vi "Continued Fraction Complex.vi"(1 "b":cdb[](array[numeric]) format="%0.2f", 2 "a":cdb[](array[numeric]) format="%0.2f") -> (0 "result":cdb format="%0.2f")   [LabVIEW 2018, in "NI_Gmath.lvlib"]
uses:
  NI_Gmath.lvlib
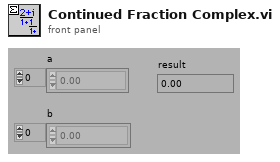
[diagram p1: front panel]
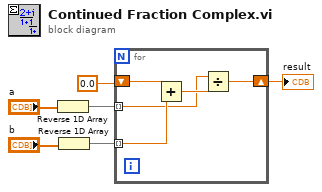
[diagram p0: block diagram]
diagram:
  n1 = Reverse 1D Array(array="a") -> (reversed array=w2:cdb[])
  n2 = Reverse 1D Array(array="b") -> (reversed array=w3:cdb[])
  n3 = for {
    shift-right: [w8] -> w1
    shift-left: 0.0 -> [w11]
    tunnel: w3 -> [w10] mode=indexing
    tunnel: w2 -> [w7] mode=indexing
    n4 = Add(x=w11, y=w10) -> (x+y=w9:cdb)
    n5 = Divide(x=w7, y=w9) -> (x/y=w8:cdb)
  }
  "result" <- w1
